vi "Variable Reference to URL.vi"(8 "error in (no error)":errorcluster, 10 "URL type":T1=enum."HiHi", 11 "variable reference":refnum<k21>="\\\\.\\sv_alarm_example\\my_number") -> (0 "error out":errorcluster, 3 "URL":string="ni.var.psp://localhost/sv_alarm_example/my_number/Alarms/HiHi/level")   [LabVIEW 2018, in "Dynamic Shared Variables.lvlib"]
doc: "Returns desired URL based on the variable reference and the type of URL desired (e.g. the tag data, HiHi, LoLo)"
uses:
  Dynamic Shared Variables.lvlib
  URL Type Enum.ctl
panel:
  out "variable reference out":refnum<k21>="\\\\.\\sv_alarm_example\\my_number"
  out "match + rest of string":string="sv_alarm_example\\my_number"
  out "string":string="\\\\.\\sv_alarm_example\\my_number"
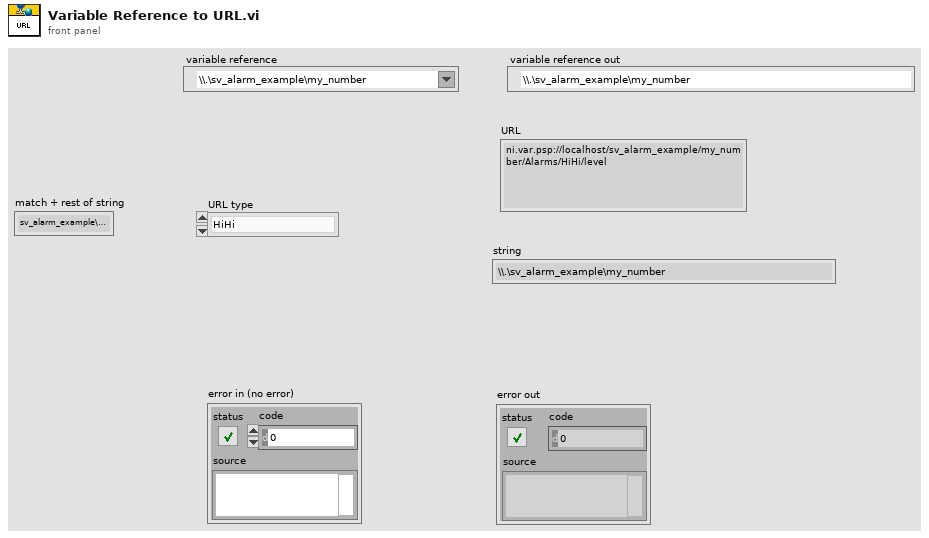
[diagram p1: front panel]
types:
  T1 = typedef "Dynamic Shared Variables.lvlib/URL Type Enum.ctl" = enum16{"Tag", "HiHi", "Hi", "Lo", "LoLo", "Tag (Bool)"}
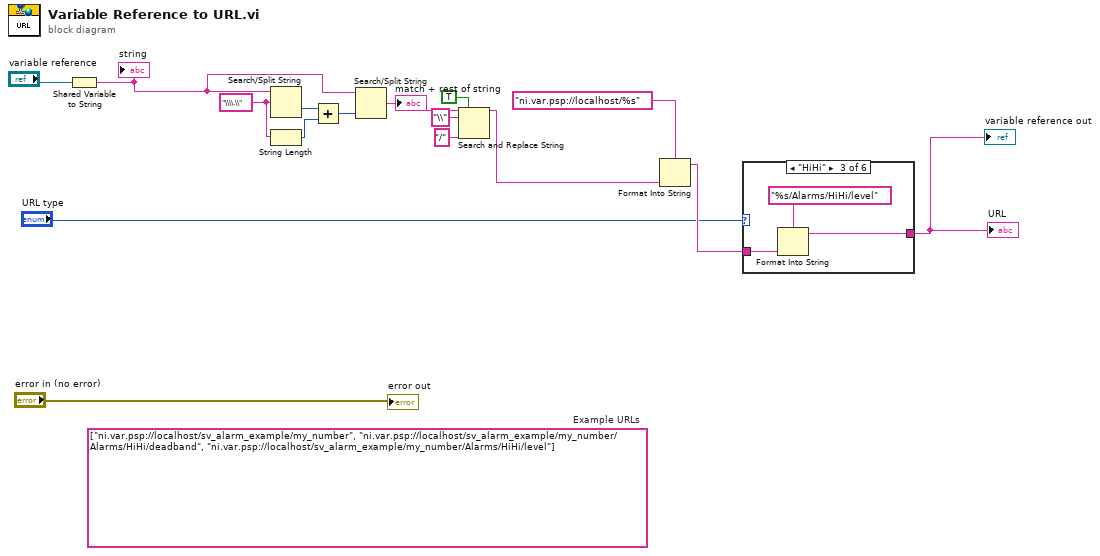
[diagram p0: block diagram]
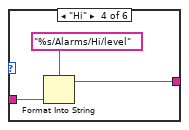
[diagram p4: hidden frame]
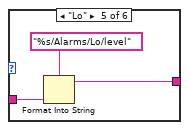
[diagram p5: hidden frame]
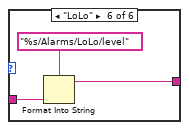
[diagram p6: hidden frame]
diagram:
  (unwired) string[] ["ni.var.psp://localhost/sv_alarm_example/my_number", "ni.var.psp://localhost/sv_alarm_example/my_number/Alarms/HiHi/deadband", "ni.var.psp://localhost/sv_alarm_example/my_number/Alarms/HiHi/level"]  # Example URLs
  w14 = "\\\\.\\" ("search string/char (-)")
  n1 = Shared Variable to String(1:"variable reference") -> (0:w15:string)
  "string" <- w15
  n2 = Search/Split String(string=w15, search string/char (-)=w14) -> (offset of match=w13:i32)  [unwired: 1 in, 2 out]
  n3 = String Length(string=w14) -> (length=w11:i32)
  n4 = Add(x=w13, y=w11) -> (x+y=w12:i32)
  n5 = Search/Split String(string=w15, offset (0)=w12) -> (match + rest of string=w10:string)  [unwired: 1 in, 2 out]
  "match + rest of string" <- w10
  n6 = Search and Replace String(replace all?=TRUE ("replace all? (F)"), input string=w10, search string="\\", replace string="/" ("replace string (\"\")")) -> (result string=w6:string)  [unwired: 4 in, 3 out]
  n7 = Format Into String(format string="ni.var.psp://localhost/%s", w6) -> (resulting string=w4:string)  [unwired: 2 in, 1 out]
  n8 = case shown="\"HiHi\"" "URL type" {
    tunnel: [w17 w18 w20 w23 w26 w29] -> w2
    tunnel: w4 -> [w17 w18 w19 w22 w25 w28]
    frame "Tag" {
    }
    frame "Tag (Bool)" {
    }
    frame "HiHi" {
      n9 = Format Into String(format string="%s/Alarms/HiHi/level", w19) -> (resulting string=w20:string)  [unwired: 2 in, 1 out]
    }
    frame "Hi" {
      n10 = Format Into String(format string="%s/Alarms/Hi/level", w22) -> (resulting string=w23:string)  [unwired: 2 in, 1 out]
    }
    frame "Lo" {
      n11 = Format Into String(format string="%s/Alarms/Lo/level", w25) -> (resulting string=w26:string)  [unwired: 2 in, 1 out]
    }
    frame "LoLo" {
      n12 = Format Into String(format string="%s/Alarms/LoLo/level", w28) -> (resulting string=w29:string)  [unwired: 2 in, 1 out]
    }
  }
  "URL" <- w2
  "variable reference out" <- w2
  "error out" <- "error in (no error)"
